vi "Data To SingleElementsArray_with_itself_csm.vi"(6 "Seperator(/)":string="/", 8 "error in (no error)":errorcluster, 10 "parentUrl":string, 11 "Cluster":variant) -> (0 "error out":errorcluster, 2 "Full NameList":string[](array[string]), 3 "DataElementArray":variant[](array[variant]))   [LabVIEW 2017, in "API String Arguments Support.lvlib"]
doc: "This VI converts a Cluster to a DataElementArray with each elements specified by parentUrl and Seperator in the form of Tree Description."
uses:
  API String Arguments Support.lvlib
  <userlib>/_NEVSTOP/Communicable State Machine(CSM)/Communicable State Machine.lvlib
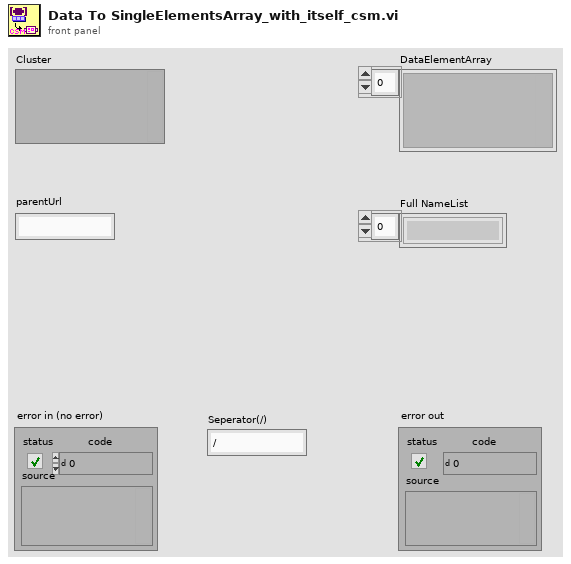
[diagram p1: front panel]
types:
  T1 = cluster{"length":u16, "private":u8, "type":enum8{"<Null>", "I8", "I16", "I32", "I64", "U8", "U16", "U32", "U64", "SGL", "DBL", "EXT", "CSG", "CDB", "CXT", "0x0F", "0x10", "0x11", "0x12", "0x13", "0x14", "Enum U8", "Enum U16", "Enum U32", "Enum U64", "SGL PQ", "DBL PQ", "EXT PQ", "CSG PQ", "CDB PQ", "CXT PQ", "0x1F", "0x20", "Boolean", "0x22", "0x23", "0x24", "0x25", "0x26", "0x27", "0x28", "0x29", "0x2A", "0x2B", "0x2C", "0x2D", "0x2E", "0x2F", "String", "0x31", "Path", "Pict", "0x34", "0x35", "0x36", "DAQ", "0x38", "0x39", "0x3A", "0x3B", "0x3C", "0x3D", "0x3E", "0x3F", "Array", "0x41", "0x42", "0x43", "0x44", "0x45", "0x46", "0x47", "0x48", "0x49", "0x4A", "0x4B", "0x4C", "0x4D", "0x4E", "0x4F", "Cluster", "0x51", "0x52", "Variant", "Waveform", "0x55", "0x56", "0x57", "0x58", "0x59", "0x5A", "0x5B", "0x5C", "0x5D", "0x5E", "Fixed Point", "0x60", "0x61", "0x62", "0x63", "0x64", "0x65", "0x66", "0x67", "0x68", "0x69", "0x6A", "0x6B", "0x6C", "0x6D", "0x6E", "0x6F", "Refnum", "0x71", "0x72", "Set Collection", "Map Collection"}, "# elements":u16}
  T2 = enum8{"<Null>", "I8", "I16", "I32", "I64", "U8", "U16", "U32", "U64", "SGL", "DBL", "EXT", "CSG", "CDB", "CXT", "0x0F", "0x10", "0x11", "0x12", "0x13", "0x14", "Enum U8", "Enum U16", "Enum U32", "Enum U64", "SGL PQ", "DBL PQ", "EXT PQ", "CSG PQ", "CDB PQ", "CXT PQ", "0x1F", "0x20", "Boolean", "0x22", "0x23", "0x24", "0x25", "0x26", "0x27", "0x28", "0x29", "0x2A", "0x2B", "0x2C", "0x2D", "0x2E", "0x2F", "String", "0x31", "Path", "Pict", "0x34", "0x35", "0x36", "DAQ", "0x38", "0x39", "0x3A", "0x3B", "0x3C", "0x3D", "0x3E", "0x3F", "Array", "0x41", "0x42", "0x43", "0x44", "0x45", "0x46", "0x47", "0x48", "0x49", "0x4A", "0x4B", "0x4C", "0x4D", "0x4E", "0x4F", "Cluster", "0x51", "0x52", "Variant", "Waveform", "0x55", "0x56", "0x57", "0x58", "0x59", "0x5A", "0x5B", "0x5C", "0x5D", "0x5E", "Fixed Point", "0x60", "0x61", "0x62", "0x63", "0x64", "0x65", "0x66", "0x67", "0x68", "0x69", "0x6A", "0x6B", "0x6C", "0x6D", "0x6E", "0x6F", "Refnum", "0x71", "0x72", "Set Collection", "Map Collection"}
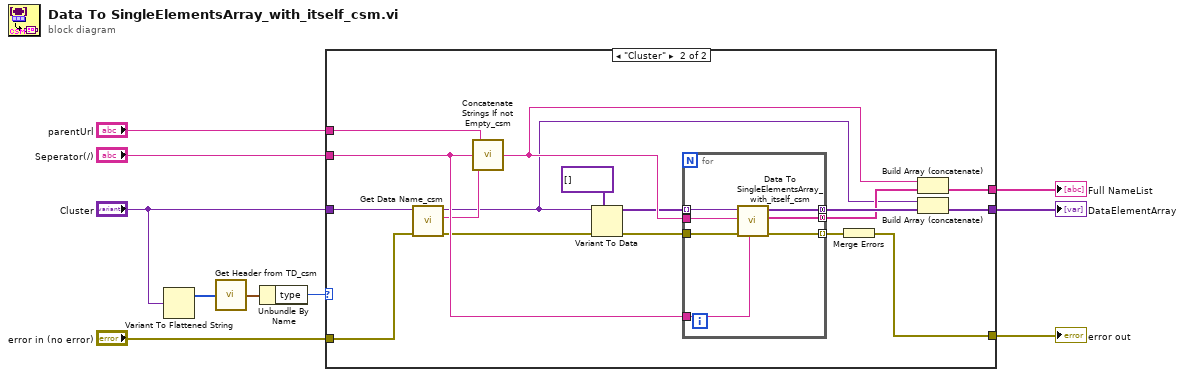
[diagram p0: block diagram]
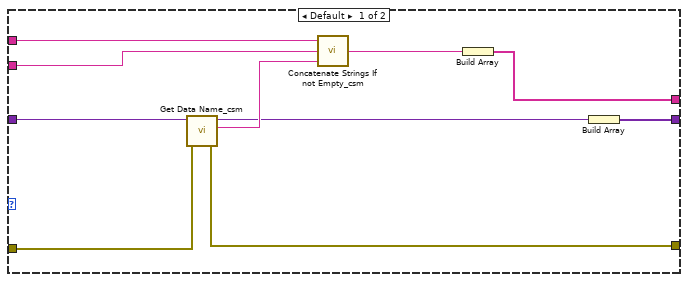
[diagram p2: hidden frame]
diagram:
  n1 = Variant To Flattened String(Variant="Cluster") -> (1:w4:i16[])  [unwired: 1 out]
  n2 = call <userlib>:"Get Header from TD_csm.vi"("Type Descriptor"=w4) -> ("Type Descriptor Header"=w3:T1)
  n3 = Unbundle By Name(w3) -> ("type"=w2:T2)
  n4 = case shown="\"Cluster\"" w2 {
    tunnel: "Cluster" -> [w20 w37]
    tunnel: "parentUrl" -> [w19 w34]
    tunnel: "error in (no error)" -> [w17 w30]
    tunnel: [w13 w35] -> w8
    tunnel: [w16 w27] -> w7
    tunnel: [w14 w31] -> w6
    tunnel: "Seperator(/)" -> [w11 w29]
    frame Default {
      n5 = call <userlib>:"Get Data Name_csm.vi"("error in (no error)"=w17, "Data"=w20) -> ("error out"=w13:errorcluster, "Data Name"=w18:string, "Data dup"=w12:variant)  [unwired: 7 in]
      n6 = call "Concatenate Strings If not Empty_csm.vi"("String"=w18, "seperator(:)"=w11, "prefix"=w19) -> ("result"=w15:string)  [unwired: 2 in]
      n7 = Build Array(w15) -> (w14:string[])
      n8 = Build Array(w12) -> (w16:variant[])
    }
    frame "Cluster" {
      n9 = call <userlib>:"Get Data Name_csm.vi"("error in (no error)"=w30, "Data"=w37) -> ("error out"=w22:errorcluster, "Data Name"=w28:string, "Data dup"=w23:variant)  [unwired: 7 in]
      n10 = call "Concatenate Strings If not Empty_csm.vi"("String"=w28, "seperator(:)"=w29, "prefix"=w34) -> ("result"=w26:string)  [unwired: 2 in]
      n11 = Variant To Data(error in=w22, type=variant[] [] ("Array"), Variant=w23) -> (data=w24:variant[], error out=w21:errorcluster)
      n12 = for {
        tunnel: w24 -> [w44] mode=indexing
        tunnel: w26 -> [w43]
        tunnel: [w42] -> w33 mode=concatenating
        tunnel: w21 -> [w41]
        tunnel: [w40] -> w36 mode=indexing
        tunnel: [w39] -> w32 mode=concatenating
        tunnel: w29 -> [w38]
        n13 = call "Data To SingleElementsArray_with_itself_csm.vi"("Seperator(/)"=w38, "error in (no error)"=w41, "parentUrl"=w43, "Cluster"=w44) -> ("error out"=w40:errorcluster, "Full NameList"=w39:string[], "DataElementArray"=w42:variant[])  [unwired: 5 in]
      }
      n14 = Merge Errors(w36) -> (w35:errorcluster)
      n15 = Build Array (concatenate)(w26, w32) -> (w31:string[])
      n16 = Build Array (concatenate)(w23, w33) -> (w27:variant[])
    }
  }
  "Full NameList" <- w6
  "error out" <- w8
  "DataElementArray" <- w7
